vi "Initialize.vi"(8 "error in (no error)":errorcluster, 11 "Scanner Port":string) -> (0 "error out":errorcluster, 3 "Scanner reference":refnum<visa-resource-name>)   [LabVIEW 2023, in "HoneywellScanner.lvlib"]
uses:
  HoneywellScanner.lvlib
  <vilib>/Instr/_visa.llb/VISA Configure Serial Port (Instr).vi
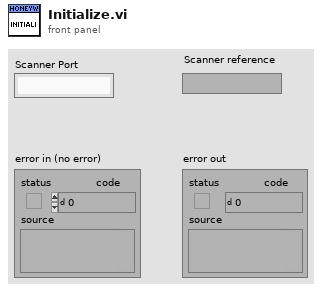
[diagram p1: front panel]
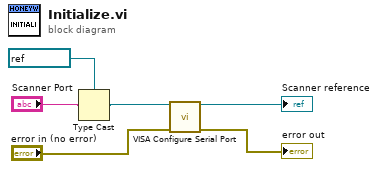
[diagram p0: block diagram]
diagram:
  n1 = Type Cast(type=refnum<visa-resource-name> "COM1" ("VISA resource name"), x="Scanner Port") -> (*(type *) &x=w5:refnum<visa-resource-name>)
  n2 = call-poly "VISA Configure Serial Port"("VISA resource name"=w5, "error in (no error)"="error in (no error)") -> ("VISA resource name out"=→"Scanner reference":refnum<visa-resource-name>, "error out"=→"error out":errorcluster)  [unwired: 12 in]
